vi "Check If Validation Needed.vi"(8 "error in (no error)":errorcluster, 10 "Module Information in":T1[](array[typedef])) -> (0 "error out":errorcluster, 1 "Needs Validation":bool, 2 "Module Information out":T1[](array[typedef]))   [LabVIEW 2020, in "Routing and Faulting System Explorer.lvlib"]
uses:
  Routing and Faulting System Explorer.lvlib
  Scripting/Types/Module Information.ctl
  Shared/Routing and Faulting Hardware API/Types/Possible Connections for Endpoint.ctl
  Shared/Routing and Faulting Hardware API/Routing and Faulting Hardware API.lvlib
  Scripting/Routing and Faulting Scripting.lvlib
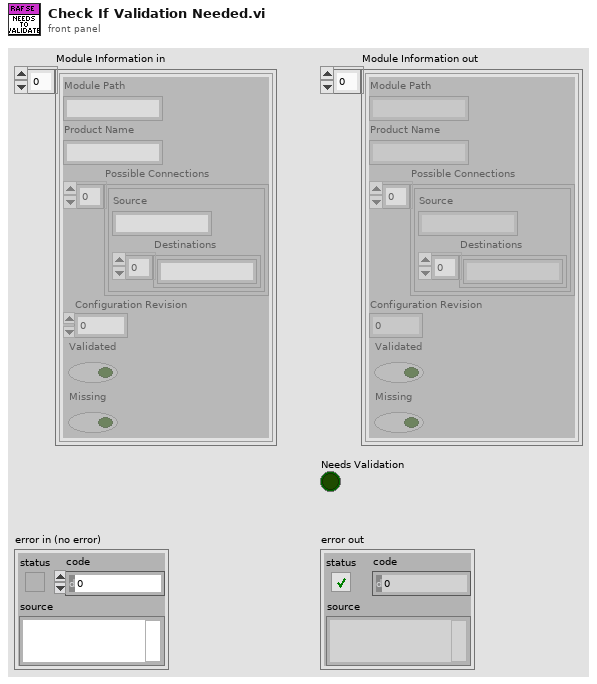
[diagram p1: front panel]
types:
  T1 = typedef "Routing and Faulting Scripting.lvlib/Module Information.ctl" = cluster{"Module Path":string, "Product Name":string, "Possible Connections":T2[], "Configuration Revision":u32, "Validated":bool, "Missing":bool}
  T2 = typedef "Routing and Faulting Hardware API.lvlib/Possible Connections for Endpoint.ctl" = cluster{"Source":string, "Destinations":string[]}
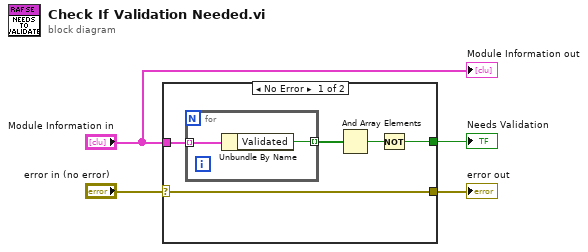
[diagram p0: block diagram]
diagram:
  n1 = case shown="No Error" "error in (no error)" {
    selector: "error in (no error)" -> [w5 w12]
    tunnel: "Module Information in" -> [w9 _]
    tunnel: [w6 _] -> w4
    tunnel: [w5 w12] -> w1
    frame No Error {
      n2 = for {
        tunnel: w9 -> [w11] mode=indexing
        tunnel: [w10] -> w8 mode=indexing
        n3 = Unbundle By Name(w11) -> ("Validated"=w10:bool)
      }
      n4 = And Array Elements(Boolean array=w8) -> (logical AND=w7:bool)
      n5 = Not(x=w7) -> (.not. x?=w6:bool)
    }
    frame Error {
    }
  }
  "Needs Validation" <- w4
  "error out" <- w1
  "Module Information out" <- "Module Information in"
